vi "slopeAtCoercivGc.vi"(8 "B":dbl[](array[numeric]), 11 "H":dbl[](array[numeric])) -> (2 "Gc":dbl)   [LabVIEW 2019]
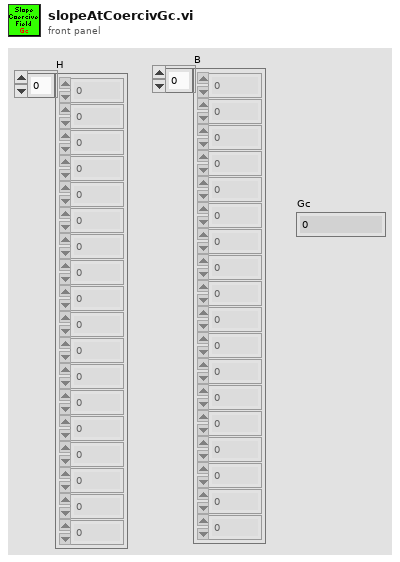
[diagram p1: front panel]
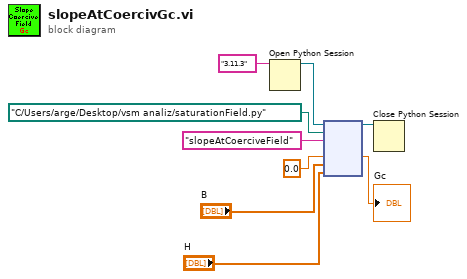
[diagram p0: block diagram]
diagram:
  n1 = Open Python Session(python version="3.11.3" ("Python version")) -> (session out=w2:refnum<k35>)  [unwired: 2 in, 1 out]
  n2 = node(w2, path "C:/Users/arge/Desktop/vsm analiz/saturationField.py" ("module path"), "slopeAtCoerciveField" ("function name"), 0.0, "B", "H") -> (w9:refnum<k35>, →"Gc":dbl)  [unwired: 3 in, 3 out]
  n3 = Close Python Session(session in=w9) -> ()  [unwired: 1 in, 1 out]
